vi "Write Object Name.vi"(8 "error in (no error)":errorcluster, 10 "Object Name":string, 11 "Detector Class in":refnum<class "Detector Class.lvclass">) -> (0 "error out":errorcluster, 3 "Detector Class out":refnum<class "Detector Class.lvclass">)   [LabVIEW 2024, in "Detector Class.lvclass"]
uses:
  Detector Class.lvclass
  Detector Class.lvclass/Detector Class.ctl
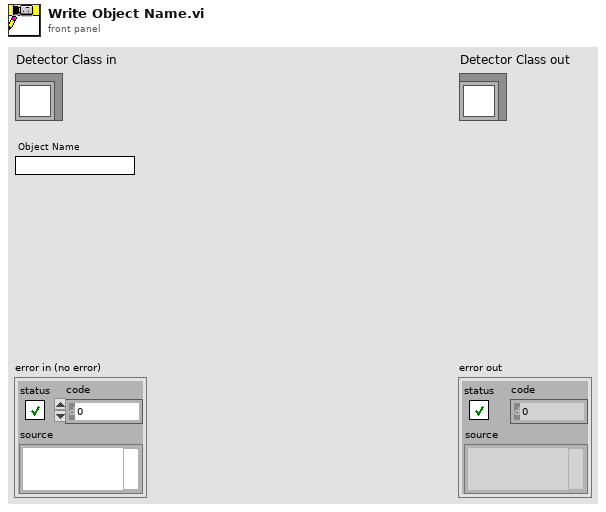
[diagram p1: front panel]
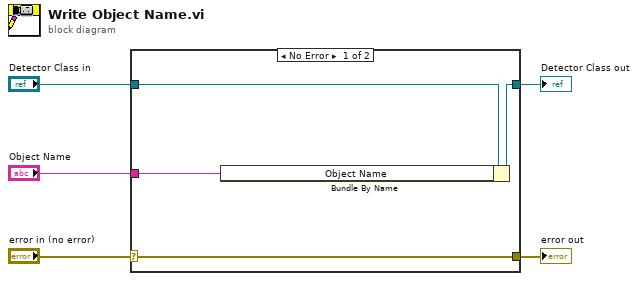
[diagram p0: block diagram]
diagram:
  n1 = case shown="No Error" "error in (no error)" {
    selector: "error in (no error)" -> [w9 w10]
    tunnel: [w9 w10] -> w4
    tunnel: [w7 w11] -> w2
    tunnel: "Detector Class in" -> [w8 w11]
    tunnel: "Object Name" -> [w6 _]
    frame No Error {
      n2 = Bundle By Name(cluster=w8, "Object Name"=w6) -> (w7:refnum<class "Detector Class.lvclass">)
    }
    frame Error {
    }
  }
  "error out" <- w4
  "Detector Class out" <- w2
